vi "LAB4-1.vi"() -> ()   [LabVIEW 2011]
uses:
  <userlib>/KNR LabVIEW Toolkit/Type Definitions/Port Number (for US).ctl
  <userlib>/KNR LabVIEW Toolkit/General/KNR Open (Direct Mode).vi
  <userlib>/KNR LabVIEW Toolkit/RC Servo Control/RC Servo Library.lvlib
  <userlib>/KNR LabVIEW Toolkit/Ultrasonic Control/Ultrasonic Library.lvlib
panel:
  in  "RC Pulse Width (uS)":u16[](array[numeric])=[1500, 1500, 1500, 1500, 1500, 1500, 1500]
  out "XY Graph":cluster{dbl[], dbl[]}(graph)
  out "Ultrasonic output":T1
  in  "Port Number":T2 items=["US1-US4"=0, "US5-US8"=2]
  in  "RC Port Power":bool
  out "error out":errorcluster
  in  "stop":bool
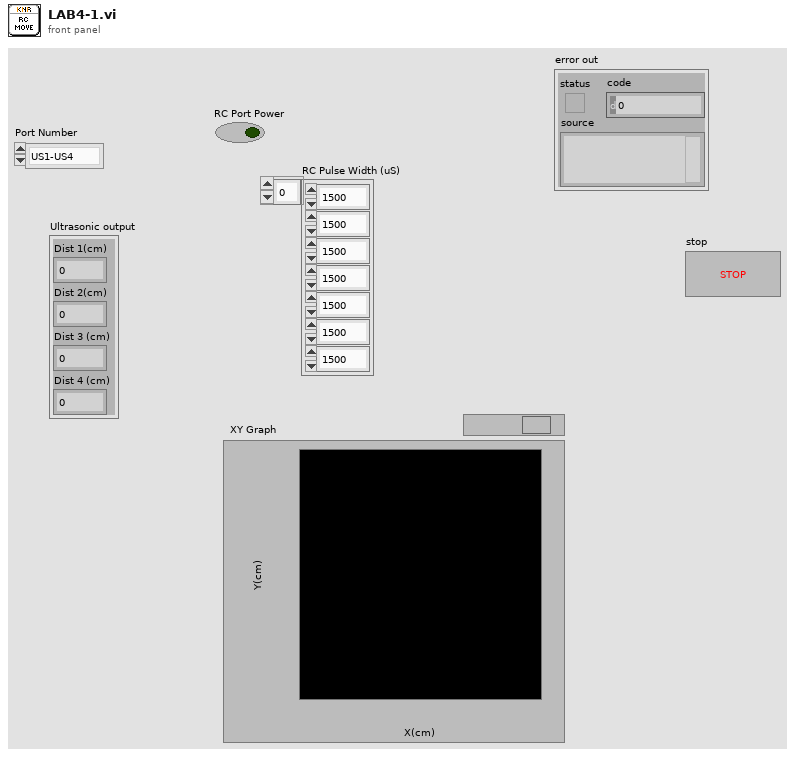
[diagram p1: front panel]
types:
  T1 = cluster{"Dist 1(cm)":dbl, "Dist 2(cm)":dbl, "Dist 3 (cm)":dbl, "Dist 4 (cm)":dbl}
  T2 = typedef "Port Number (for US).ctl" = u16
  T3 = typedef "KNR Reference.ctl" = cluster{"FPGA Session":refnum<class "FPGA Interface Base.lvclass">, "Port Types":T4[]}
  T4 = typedef "Port Type (API).ctl" = enum8{"Unassigned", "DIO", "DC Motor", "RC Motor", "Ultrasonic", "Analog Input"}
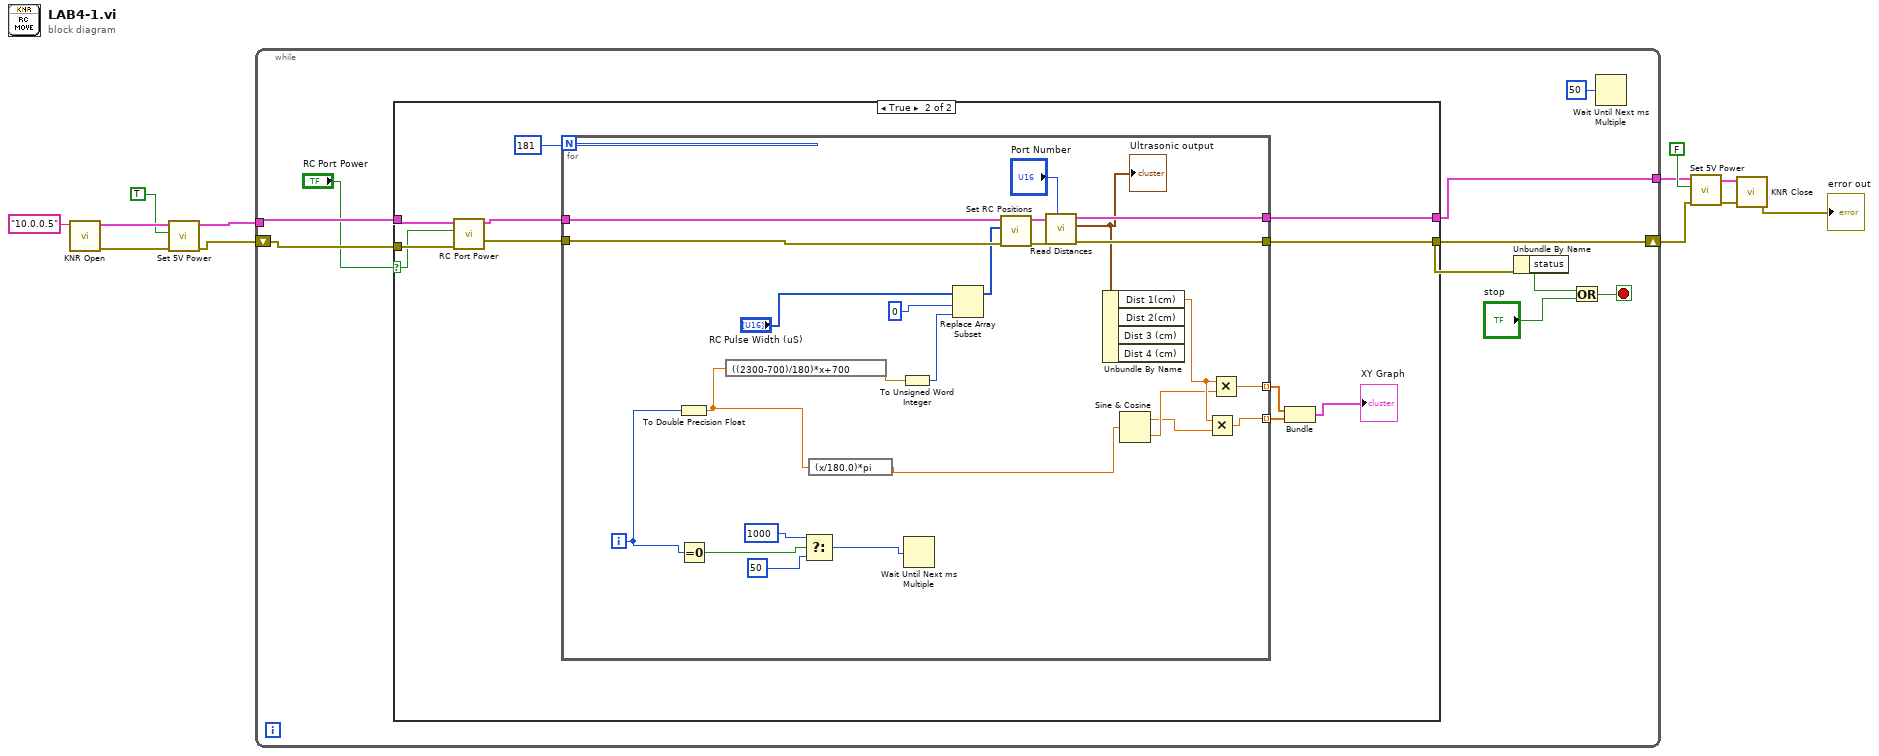
[diagram p0: block diagram]
diagram:
  n1 = call-poly <userlib>:"KNR Open.vi"("IP Address (Default: 10.0.0.5)"="10.0.0.5") -> ("error out"=w11:errorcluster, "KNR Out"=w12:T3)  [unwired: 9 in]
  n2 = call <userlib>:"Set 5V Power.vi"("error in (no error)"=w11, "5V Power"=TRUE, "KNR In"=w12) -> ("error out"=w1:errorcluster, "KNR Out"=w9:T3)  [unwired: 7 in]
  n3 = while {
    tunnel: w9 -> [w18]
    tunnel: [w15] -> w2
    shift-right: [w17] -> w3
    shift-left: w1 -> [w14]
    stop <- w20 stop-if-true
    n4 = case shown="True" "RC Port Power" {
      selector: "RC Port Power" -> [_ w24]
      tunnel: w18 -> [w23 w34]
      tunnel: [w22 w31] -> w17
      tunnel: [w23 w26] -> w15
      tunnel: w14 -> [w22 w25]
      frame False {
      }
      frame True {
        n5 = call <userlib>:"RC Port Power.vi"("error in (no error)"=w25, "RC Power"=w24, "KNR In"=w34) -> ("error out"=w32:errorcluster, "KNR Out"=w33:T3)  [unwired: 7 in]
        n6 = for {
          N: 181 -> [_]
          tunnel: w33 -> [w59]
          tunnel: w32 -> [w58]
          tunnel: [w54] -> w26
          tunnel: [w53] -> w31
          tunnel: [w48] -> w29 mode=indexing
          tunnel: [w47] -> w28 mode=indexing
          i -> [w35]
          n7 = To Double Precision Float(number=w35) -> (double precision float=w42:dbl)
          n8 = Equal To 0?(x=w35) -> (x = 0?=w36:bool)
          n9 = expression code="((2300-700)/180)*x+700"(w42) -> (w40:dbl)
          n10 = Select(t=1000, s=w36, f=50) -> (s? t:f=w46:i32)
          n11 = expression code="(x/180.0)*pi"(w42) -> (w43:dbl)
          n12 = To Unsigned Word Integer(number=w40) -> (unsigned 16bit integer=w39:u16)
          n13 = Wait Until Next ms Multiple(millisecond multiple=w46) -> ()  [unwired: 1 out]
          n14 = Replace Array Subset(array="RC Pulse Width (uS)", new element=w39, index=0) -> (w38:u16[])
          n15 = call <userlib>:"Set RC Positions.vi"("error in (no error)"=w58, "RC Pulse Width (uS)"=w38, "KNR In"=w59) -> ("error out"=w55:errorcluster, "KNR Out"=w56:T3)  [unwired: 7 in]
          n16 = call <userlib>:"Read Distances.vi"("Port Number"="Port Number", "error in (no error)"=w55, "KNR In"=w56) -> ("error out"=w53:errorcluster, "Ultrasonic output"=w52:T1, "KNR Out"=w54:T3)  [unwired: 6 in]
          "Ultrasonic output" <- w52
          n17 = Unbundle By Name(w52) -> ("Dist 1(cm)"=w51:dbl)  [unwired: 3 out]
          n18 = Sine & Cosine(0:w43) -> (1:w49:dbl, 2:w50:dbl)
          n19 = Multiply(x=w51, y=w49) -> (x*y=w47:dbl)
          n20 = Multiply(x=w51, y=w50) -> (x*y=w48:dbl)
        }
        n21 = Bundle(w29, w28) -> (→"XY Graph":cluster{dbl[], dbl[]})  [unwired: 1 in]
      }
    }
    n22 = Unbundle By Name(w17) -> ("status"=w16:bool)
    n23 = Or(x=w16, y="stop") -> (x .or. y?=w20:bool)
    n24 = Wait Until Next ms Multiple(millisecond multiple=u32 50) -> ()  [unwired: 1 out]
  }
  n25 = call <userlib>:"Set 5V Power.vi"("error in (no error)"=w3, "5V Power"=FALSE, "KNR In"=w2) -> ("error out"=w4:errorcluster, "KNR Out"=w6:T3)  [unwired: 7 in]
  n26 = call <userlib>:"KNR Close.vi"("error in (no error)"=w4, "KNR In"=w6) -> ("error out"=→"error out":errorcluster)  [unwired: 9 in]
